vi "Practica 2.vi"() -> ()   [LabVIEW 2018]
panel:
  out "Numeric 4":dbl
  in  "Joules":dbl
  out "Frecuencia 1":dbl
  in  "Longitud 1":dbl
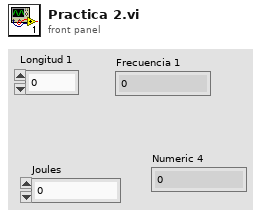
[diagram p1: front panel]
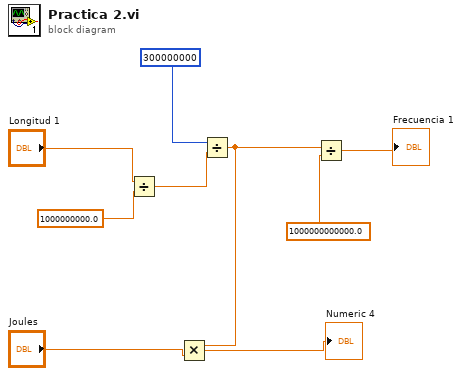
[diagram p0: block diagram]
diagram:
  n1 = Divide(x="Longitud 1", y=1000000000.0) -> (x/y=w6:dbl)
  n2 = Divide(x=300000000, y=w6) -> (x/y=w2:dbl)
  n3 = Multiply(x=w2, y="Joules") -> (x*y=→"Numeric 4":dbl)
  n4 = Divide(x=w2, y=1000000000000.0) -> (x/y=→"Frecuencia 1":dbl)
